vi "tryRead.vi"(8 "error in (no error)":errorcluster, 11 "Communicator in":refnum<class "Communicator.lvclass">) -> (0 "error out":errorcluster, 2 "Message":T1, 3 "Communicator out":refnum<class "Communicator.lvclass">)   [LabVIEW 2016]
uses:
  Communicator.lvclass
  DataTypes/MessageTypes.ctl
  M1M3Communicator.lvlib
  DataTypes/MessageTopics.ctl
  DataTypes/MessageHeader.ctl
  DataTypes/Message.ctl
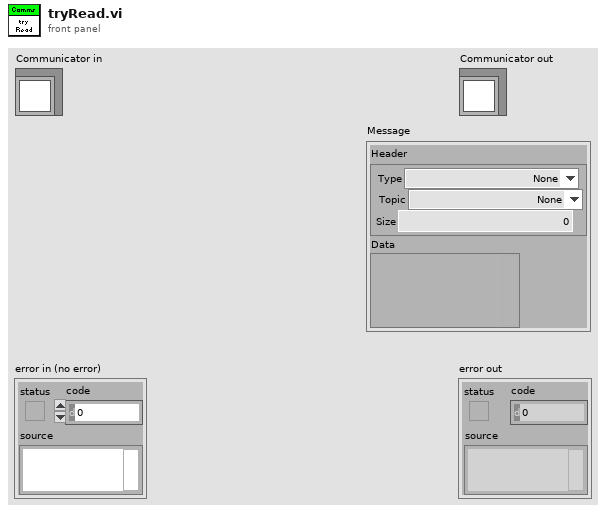
[diagram p1: front panel]
types:
  T1 = typedef "M1M3Communicator.lvlib/Message.ctl" = cluster{"Header":T2, "Data":variant}
  T2 = typedef "M1M3Communicator.lvlib/MessageHeader.ctl" = cluster{"Type":T3, "Topic":T4, "Size":i32}
  T3 = typedef "M1M3Communicator.lvlib/MessageTypes.ctl" = enum8{"None", "PutSample", "GetNextSample", "LogEvent", "GetEvent", "IssueCommand", "CommandId", "WaitForCompletion", "AcceptCommand", "AckCommand"}
  T4 = typedef "M1M3Communicator.lvlib/MessageTopics.ctl" = enum8{"None", "Start", "Enable", "Disable", "Standby", "AppliedSettingsMatchStart", "ErrorCode", "SettingVersions", "SummaryState", "DetailedState", "Exit"}
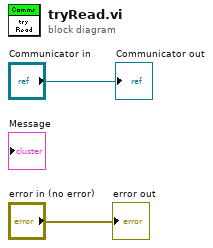
[diagram p0: block diagram]
diagram:
  "error out" <- "error in (no error)"
  "Communicator out" <- "Communicator in"
